vi "File FGV.vi"(9 "데이터":dbl[][](array[numeric]), 10 "파일 경로":path, 11 "File FGV 상태":enum16{"열기", "쓰기", "닫기"}(ring)) -> ()   [LabVIEW 2020]
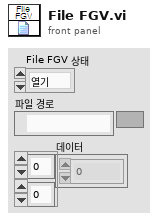
[diagram p1: front panel]
types:
  T1 = enum16{"open", "open or create", "create or replace", "create", "open (read-only)"}
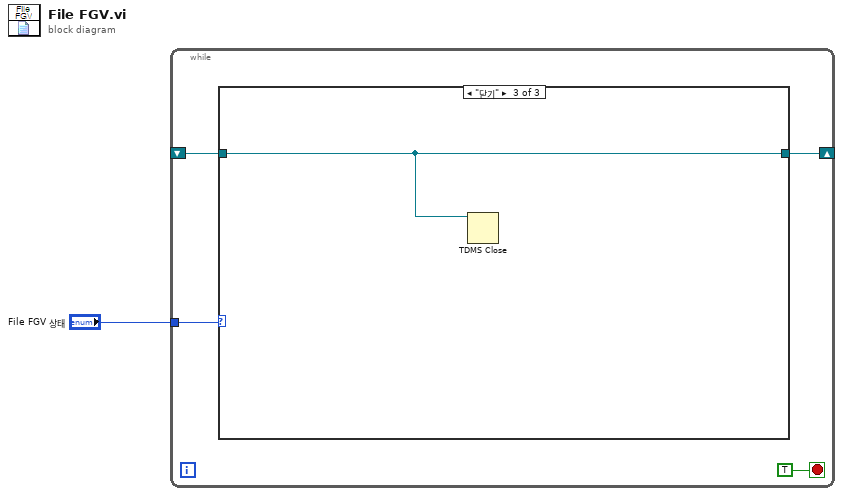
[diagram p0: block diagram]
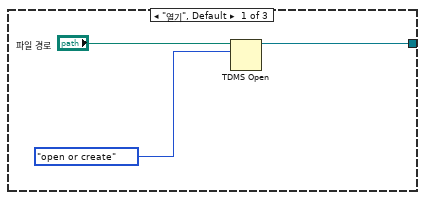
[diagram p2: hidden frame]
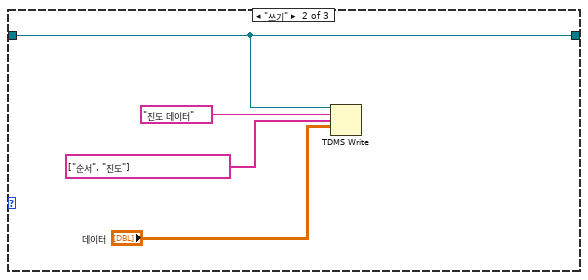
[diagram p3: hidden frame]
diagram:
  n1 = while {
    shift-right: [w3] -> _
    shift-left: _ -> [w2]
    tunnel: "File FGV 상태" -> [w4]
    stop <- TRUE stop-if-true
    n2 = case shown="\"닫기\"" w4 {
      tunnel: [w8 w12 w13] -> w3
      tunnel: w2 -> [_ w12 w13]
      frame "열기", Default {
        n3 = TDMS Open(10:T1."open or create" ("동작(0:open)"), 11:"파일 경로") -> (3:w8:refnum<k34>)  [unwired: 5 in, 1 out]
      }
      frame "쓰기" {
        n4 = TDMS Write(0:w12, 5:"진도 데이터", 7:string[] ["순서", "진도"], 9:"데이터") -> ()  [unwired: 2 in, 4 out]
      }
      frame "닫기" {
        n5 = TDMS Close(11:w13) -> ()  [unwired: 1 in, 2 out]
      }
    }
  }
